vi "ATF-Pump-Data Transfer Loop RD.vi"(11 "Data FIFO Ref":T1) -> ()   [LabVIEW 2022 SP3]
uses:
  RT Controls/ATF-Pump-Data FIFO.ctl
  RT Controls/ATF-Pump-DiplayPC comm ctrl.ctl
  <vilib>/Platform/TimedLoop/XDataNode/timing_clust.ctl
  <vilib>/Platform/TimedLoop/XDataNode/nitl_modes.ctl
  <vilib>/Platform/TimedLoop/XDataNode/wakeup.ctl
  RT Support/ATF-Pump-RT_Global_R.vi
  <vilib>/platform/TimedLoop/XDataNode/XDataNode.xnode
  <vilib>/Platform/TimedLoop/XDataNode/XDNodeRunTimeDep.lvlib
panel:
  out "length":i32
  out "x-y":u32
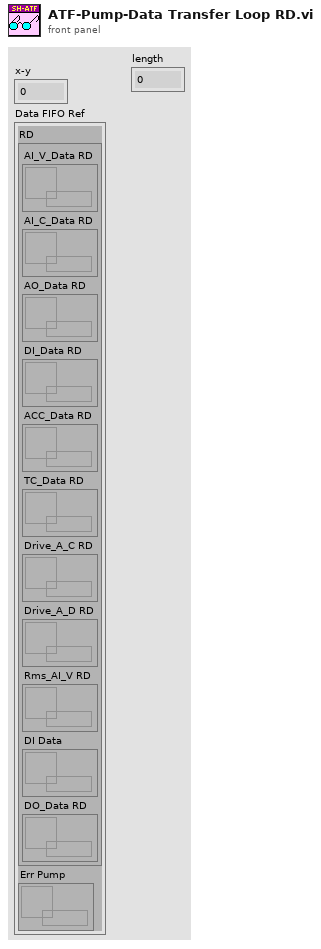
[diagram p1: front panel]
types:
  T1 = typedef "ATF-Pump-Data FIFO.ctl" = cluster{"RD":cluster{"AI_V_Data RD":refnum<queue>, "AI_C_Data RD":refnum<queue>, "AO_Data RD":refnum<queue>, "DI_Data RD":refnum<queue>, "ACC_Data RD":refnum<queue>, "TC_Data RD":refnum<queue>, "Drive_A_C RD":refnum<queue>, "Drive_A_D RD":refnum<queue>, "Rms_AI_V RD":refnum<queue>, "DI Data":refnum<queue>, "DO_Data RD":refnum<queue>}, "Err Pump":refnum<queue>}
  T2 = typedef "ATF-Pump-DiplayPC comm ctrl.ctl" = enum16{"Initialize", "Listen for UI Writer", "Send RT Data"}
  T3 = typedef "XDNodeRunTimeDep.lvlib/timing_clust.ctl" = cluster{"Expected End [f-1]":u64, "Actual End [f-1]":u64, "Finished Late? [f-1]":bool, "Expected End [i-1]":u64, "Actual End [i-1]":u64, "Finished Late? [i-1]":bool, "Expected Start [i]":u64, "Actual Start [i]":u64, "Expected Start [f]":u64, "Actual Start [f]":u64, "Source Name":string, "Structure Name":string, "Period":i64, "Deadline":i64, "Offset":i64, "Start":i64, "Priority":i32, "Timeout":i32, "Mode":T4, "Wakeup Reason":T5, "Error":errorcluster, "Source Type":string, "Secondary Source Type":string, "Global End Time":u64, "Global Start Time":u64, "Frame Duration":u64, "Iteration Duration":u64, "Assigned CPU":i32, "I/O Scan Engine Mode":u32}
  T4 = typedef "XDNodeRunTimeDep.lvlib/nitl_modes.ctl" = enum32{"No Change", "Process missed periods, maintain original phase", "Discard missed periods, maintain original phase", "Process missed periods, ignore original phase", "Discard missed periods, ignore original phase"}
  T5 = typedef "XDNodeRunTimeDep.lvlib/wakeup.ctl" = enum32{"Normal", "Aborted", "Asynchronous wakeup", "Timing source error", "Timed loop error", "Timeout"}
  T6 = cluster{"Start DAQ":bool, "Stop DAQ":bool, "RT Stop":bool, "RT Exit":bool, "Start Seq":bool}
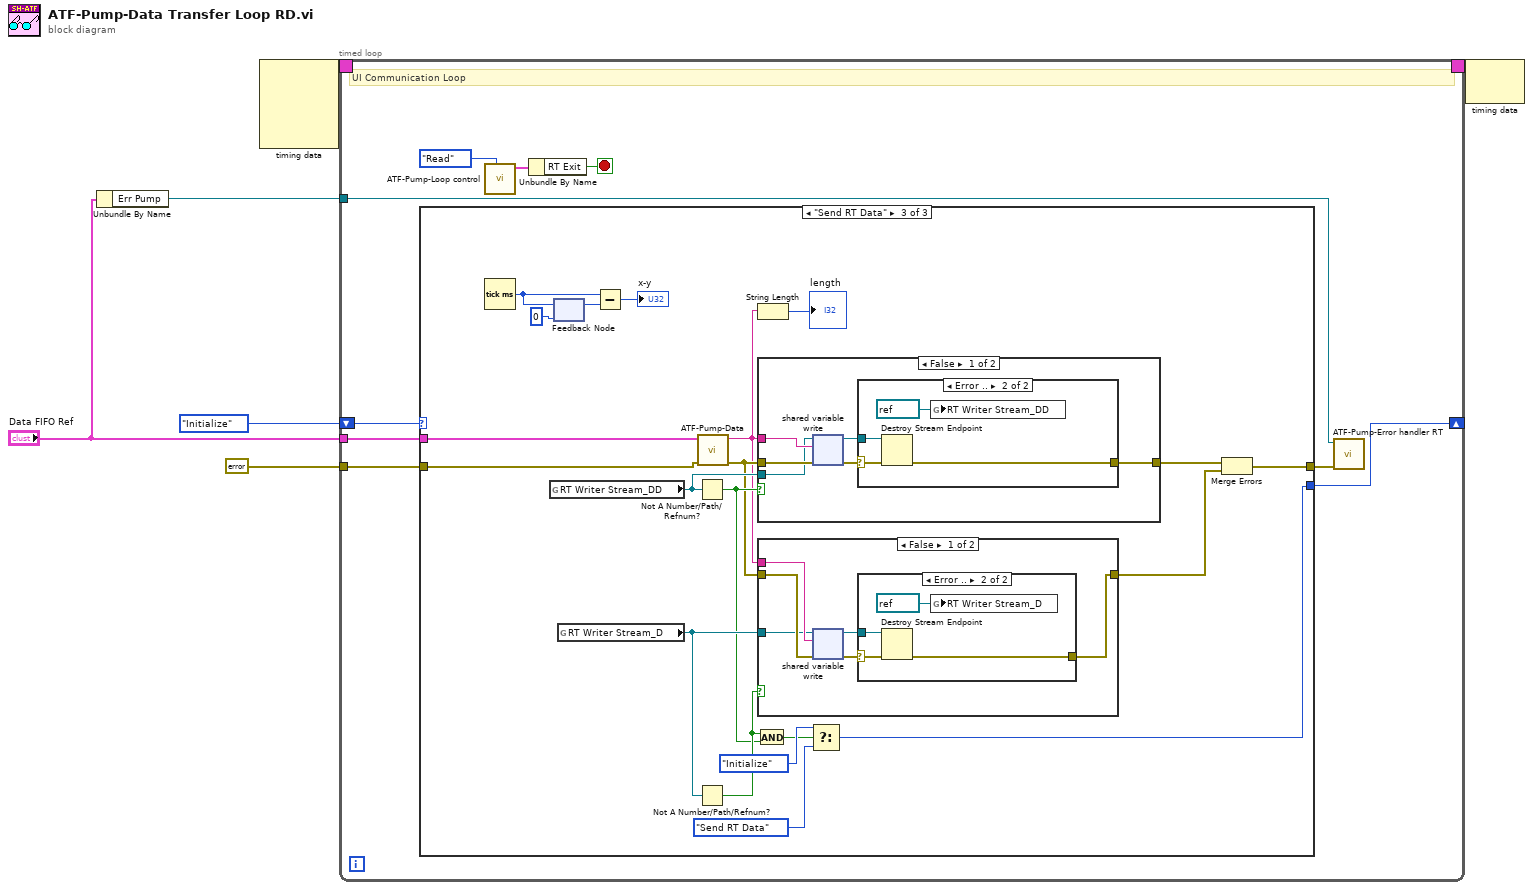
[diagram p0: block diagram]
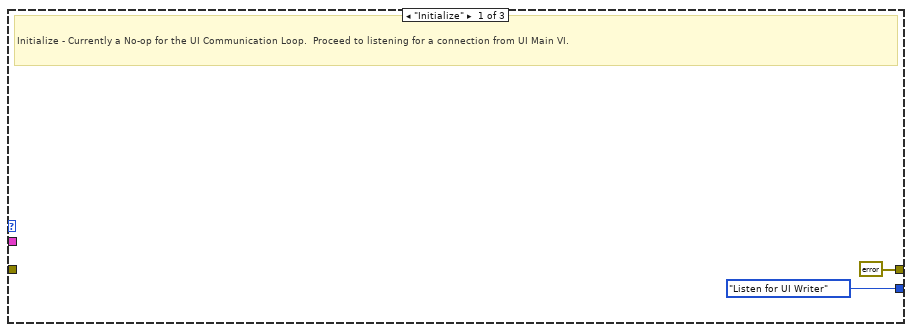
[diagram p2: hidden frame]
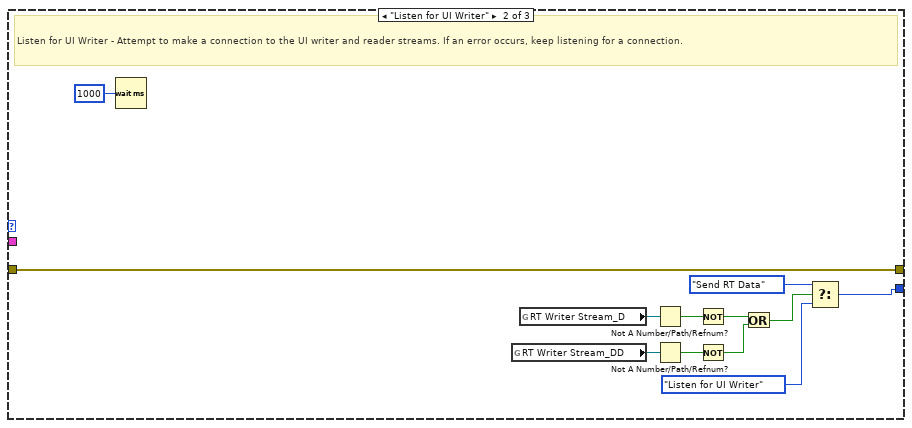
[diagram p3: hidden frame]
diagram:
  n1 = Unbundle By Name("Data FIFO Ref") -> ("Err Pump"=w1:refnum<queue>)
  n2 = node-c288() -> (w4:T3)  [unwired: 4 in]
  n3 = timed-loop {
    shift-right: [w15] -> _
    shift-left: ATF-Pump-DiplayPC_comm_ctrl."Initialize" -> [w14]
    tunnel: "Data FIFO Ref" -> [w13]
    tunnel: errorcluster {"status"=FALSE, "code"=0, "source"=""} ("error in (no error)") -> [w8]
    timing: w4 -> [_]
    timing-out: [_] -> w3
    tunnel: w1 -> [w7]
    stop <- w10 stop-if-true
    # "UI Communication Loop"
    n4 = case shown="\"Send RT Data\"" w14 {
      tunnel: [errorcluster {"status"=FALSE, "code"=0, "source"=""} ("error IO") w18 w34] -> w9
      tunnel: [ATF-Pump-DiplayPC_comm_ctrl."Listen for UI Writer" w23 w45] -> w15
      tunnel: w13 -> [_ _ w36]
      tunnel: w8 -> [_ w18 w37]
      frame "Initialize" {
        # "Initialize - Currently a No-op for the UI Communication Loop.  Proceed to listening for a connection from UI Main VI."
      }
      frame "Listen for UI Writer" {
        # "Listen for UI Writer - Attempt to make a connection to the UI writer and reader streams. If an error occurs, keep listening for a connection."
        n5 = Wait (ms)(milliseconds to wait=u32 1000) -> ()  [unwired: 1 out]
        n6 = global read "ATF-Pump-RT_Global_R.vi" "RT Writer Stream_DD"() -> (w28:refnum<k21>)
        n7 = global read "ATF-Pump-RT_Global_R.vi" "RT Writer Stream_D"() -> (w29:refnum<k21>)
        n8 = Not A Number/Path/Refnum?(number/path/refnum=w29) -> (NaN/Path/Refnum?=w27:bool)
        n9 = Not A Number/Path/Refnum?(number/path/refnum=w28) -> (NaN/Path/Refnum?=w26:bool)
        n10 = Not(x=w27) -> (.not. x?=w25:bool)
        n11 = Not(x=w26) -> (.not. x?=w24:bool)
        n12 = Or(x=w25, y=w24) -> (x .or. y?=w20:bool)
        n13 = Select(t=ATF-Pump-DiplayPC_comm_ctrl."Send RT Data", s=w20, f=ATF-Pump-DiplayPC_comm_ctrl."Listen for UI Writer") -> (s? t:f=w23:T2)
      }
      frame "Send RT Data" {
        n14 = Tick Count (ms)() -> (millisecond timer value=w42:u32)
        n15 = global read "ATF-Pump-RT_Global_R.vi" "RT Writer Stream_DD"() -> (w43:refnum<k21>)
        n16 = feedback-in #1(w42) -> ()
        n17 = feedback #1(u32 0 ("millisecond timer value")) -> (w41:u32)
        n18 = global read "ATF-Pump-RT_Global_R.vi" "RT Writer Stream_D"() -> (w49:refnum<k21>)
        n19 = Subtract(x=w42, y=w41) -> (x-y=→"x-y":u32)
        n20 = Not A Number/Path/Refnum?(number/path/refnum=w43) -> (NaN/Path/Refnum?=w38:bool)
        n21 = Not A Number/Path/Refnum?(number/path/refnum=w49) -> (NaN/Path/Refnum?=w44:bool)
        n22 = call "ATF-Pump-Data.vi"("error in (no error)"=w37, "Data FIFO Ref"=w36) -> ("error out"=w32:errorcluster, "data"=w31:string)  [unwired: 8 in]
        n23 = And(x=w44, y=w38) -> (x .and. y?=w46:bool)
        n24 = String Length(string=w31) -> (length=→"length":i32)
        n25 = case shown="False" w38 {
          tunnel: w43 -> [w50 _]
          tunnel: w32 -> [w53 w61]
          tunnel: [w52 w61] -> w39
          tunnel: w31 -> [w51 _]
          frame False {
            n26 = shared-variable-write(w50, w53, w51) -> (w54:refnum<k21>, w55:errorcluster)  [unwired: 1 in, 1 out]
            n27 = case shown="Error .." w55 {
              selector: w55 -> [w56 w59]
              tunnel: w54 -> [_ w60]
              tunnel: [w56 w57] -> w52
              frame No Error {
              }
              frame Error {
                n28 = Destroy Stream Endpoint(8:w59, 11:w60) -> (0:w57:errorcluster)
                n29 = global write "ATF-Pump-RT_Global_R.vi" "RT Writer Stream_DD"(refnum<k21> refnum ("RT Writer Stream_DD")) -> ()
              }
            }
          }
          frame True {
          }
        }
        n30 = case shown="False" w44 {
          tunnel: w49 -> [w62 _]
          tunnel: w32 -> [w64 w73]
          tunnel: [w65 w73] -> w33
          tunnel: w31 -> [w63 _]
          frame False {
            n31 = shared-variable-write(w62, w64, w63) -> (w66:refnum<k21>, w67:errorcluster)  [unwired: 1 in, 1 out]
            n32 = case shown="Error .." w67 {
              selector: w67 -> [w68 w71]
              tunnel: w66 -> [_ w72]
              tunnel: [w68 w69] -> w65
              frame No Error {
              }
              frame Error {
                n33 = Destroy Stream Endpoint(8:w71, 11:w72) -> (0:w69:errorcluster)
                n34 = global write "ATF-Pump-RT_Global_R.vi" "RT Writer Stream_D"(refnum<k21> refnum ("RT Writer Stream_DD")) -> ()
              }
            }
          }
          frame True {
          }
        }
        n35 = Select(t=ATF-Pump-DiplayPC_comm_ctrl."Initialize", s=w46, f=ATF-Pump-DiplayPC_comm_ctrl."Send RT Data") -> (s? t:f=w45:T2)
        n36 = Merge Errors(w39, w33) -> (w34:errorcluster)
      }
    }
    n37 = call "ATF-Pump-Loop control.vi"("Action"=enum16{"Init", "Write", "Read"}."Read") -> ("Loop Control out"=w12:T6)  [unwired: 9 in, 1 out]
    n38 = Unbundle By Name(w12) -> ("RT Exit"=w10:bool)
    n39 = call "ATF-Pump-Error handler RT.vi"("error in"=w9, "Message Queue"=w7) -> ()  [unwired: 8 in, 2 out]
  }
  n40 = node-c288(w3) -> ()  [unwired: 1 out]
